vi "Init.vi"(11 "Init Cluster":T2={"Path to server"="C:\\\\ASC500\\\\Wrapper_2.7\\\\ASC500CL-16_10_25", "Server Host"=""}) -> (0 "error out":T1)   [LabVIEW 2016]
doc: "This VI establishes a connection to the server and starts a new server if none is running at that moment. The init cluster contains:\n- server path (string): Path to the file \"daisysrv.exe\". It can usually be found in the installation directory of daisy.\n- server host (string): Hostname or IP address in \"dotted decimal\" notation for the host where the application server resides. Empty if the server should run locally.\n\nIf there is no server running already, the server path specifies the location of the server executable. Server host should only be declared if you want to access a running server on a different computer."
uses:
  Controls/Init_Parameters.ctl
  Controls/Error_Out.ctl
  Files_ASC500/DLL/ASC500_RemoteControlV27.dll
panel:
  in  "Server Port":i32=7000
  in  "Application Name":string
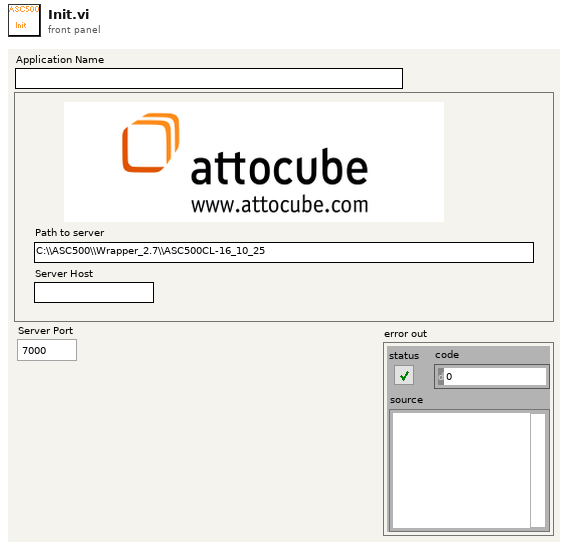
[diagram p1: front panel]
types:
  T1 = typedef "Error_Out.ctl" = errorcluster
  T2 = typedef "Init_Parameters.ctl" = cluster{"Path to server":string, "Server Host":string}
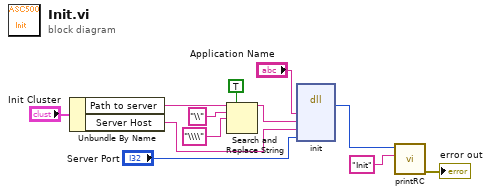
[diagram p0: block diagram]
diagram:
  n1 = Unbundle By Name("Init Cluster") -> ("Path to server"=w5:string, "Server Host"=w10:string)
  n2 = Search and Replace String(replace all?=TRUE ("replace all? (F)"), input string=w5, search string="\\", replace string="\\\\" ("search string")) -> (result string=w1:string)  [unwired: 4 in, 3 out]
  n3 = dll-call lib="G:/SCMOperations/Share/ELE/Produkt Information/ASC500/04 Remote Control/02 development versions/2018Nov06/Files_ASC500/DLL/ASC500_RemoteControlV27.dll" fn="init"("ApplicationName"="Application Name", "ServerPath"=w1, "ServerHost"=w10, "ServerPort"="Server Port") -> ("return type"=w9:i32)  [unwired: 7 in, 2 out]
  n4 = call "printRC.vi"("additional information"="Init" ("Init"), "RC"=w9) -> ("error out"=→"error out":T1)  [unwired: 9 in]
